vi "Solve1.vi"(8 "Error In":errorcluster, 11 "object in":refnum<class "2024_12.lvclass">) -> (0 "Error Out":errorcluster, 2 "Result":u64, 3 "object out":refnum<class "2024_12.lvclass">)   [LabVIEW 2023, in "2024_12.lvclass"]
uses:
  2024_12.lvclass
  2024_12.lvclass/2024_12.ctl
  f444b186-b13a-4318-b9c4-f3d0cdaa4562.vi
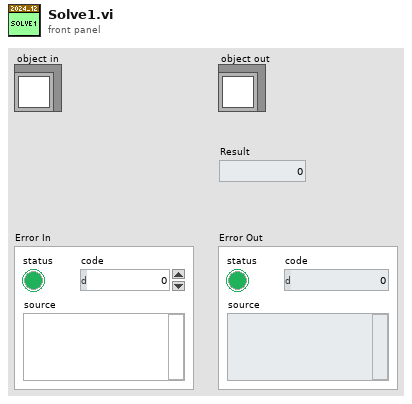
[diagram p1: front panel]
types:
  T1 = cluster{u8, cluster{i32, i32}, "PixelsFound":cluster{"x":i32, "y":i32}[]}
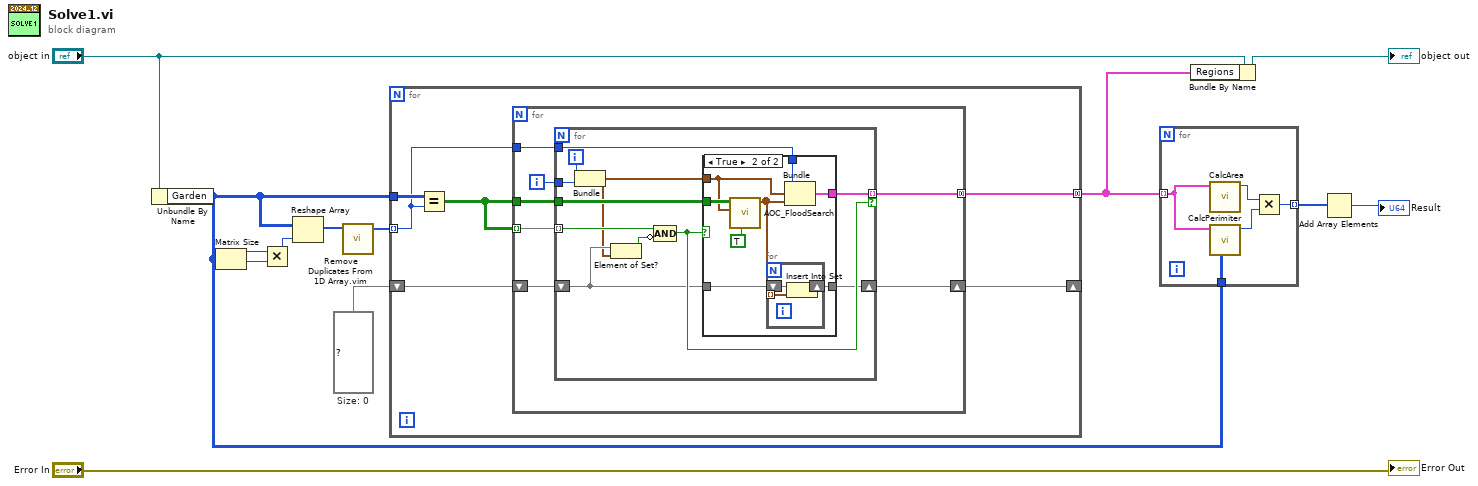
[diagram p0: block diagram]
diagram:
  w6 = set{cluster{"x":i32, "y":i32}} {}  # Size: 0
  n1 = Unbundle By Name("object in") -> ("Garden"=w3:u8[][])
  n2 = Matrix Size(0:w3) -> (1:w11:i32, 2:w10:i32)
  n3 = Multiply(x=w11, y=w10) -> (x*y=w9:i32)
  n4 = Reshape Array(w3, w9) -> (w8:u8[])
  n5 = call "Remove Duplicates From 1D Array.vim"("array"=w8) -> ("array with duplicates removed"=w7:u8[])  [unwired: 10 in]
  n6 = for {
    tunnel: w3 -> [w19]
    tunnel: w7 -> [w17] mode=indexing
    shift-right: [w15] -> _
    shift-left: w6 -> [w16]
    tunnel: [w14] -> w1 mode=concatenating
    n7 = Equal?(x=w19, y=w17) -> (x = y?=w18:bool[][])
    n8 = for {
      tunnel: w18 -> [w26]
      tunnel: w18 -> [w25] mode=indexing
      tunnel: w17 -> [w23]
      shift-right: [w21] -> w15
      shift-left: w16 -> [w22]
      tunnel: [w20] -> w14 mode=concatenating
      i -> [w24]
      n9 = for {
        tunnel: w26 -> [w37]
        tunnel: w25 -> [w36] mode=indexing
        tunnel: w24 -> [w35]
        tunnel: [w33] -> w20 mode=indexing if=w31
        tunnel: w23 -> [w32]
        shift-right: [w30] -> w21
        shift-left: w22 -> [w29]
        i -> [w34]
        n10 = Bundle(w34, w35) -> (w28:cluster{i32, i32})  [unwired: 1 in]
        n11 = Element of Set?(10:w28, 11:w29) -> (3:w27:bool)
        n12 = Compound Arithmetic op=AND(w36, invert w27) -> (w31:bool)
        n13 = case shown="True" w31 {
          tunnel: w37 -> [_ w46]
          tunnel: w28 -> [_ w45]
          tunnel: [_ w44] -> w33
          tunnel: w32 -> [_ w43]
          tunnel: w29 -> [w38 w42]
          tunnel: [w38 w41] -> w30
          frame False {
          }
          frame True {
            n14 = call "AOC_FloodSearch.vi"("4 (T) or 8 (F)"=TRUE, "Start Position"=w45, "DataIn"=w46) -> ("PixelsFound"=w40:cluster{"x":i32, "y":i32}[])  [unwired: 5 in, 3 out]
            n15 = for {
              shift-right: [w48] -> w41
              shift-left: w42 -> [w49]
              tunnel: w40 -> [w47] mode=indexing
              n16 = Insert Into Set(10:w47, 11:w49) -> (3:w48:set{cluster{"x":i32, "y":i32}})  [unwired: 1 out]
            }
            n17 = Bundle(w43, w45, "PixelsFound"=w40) -> (w44:T1)  [unwired: 1 in]
          }
        }
      }
    }
  }
  n18 = for {
    tunnel: w1 -> [w54] mode=indexing
    tunnel: [w52] -> w5 mode=indexing
    tunnel: w3 -> [w51]
    n19 = call "CalcArea.vi"("Cluster"=w54) -> ("Numeric"=w50:u64)  [unwired: 10 in]
    n20 = call "CalcPerimiter.vi"("Garden"=w51, "Cluster"=w54) -> ("Numeric"=w53:u64)  [unwired: 9 in]
    n21 = Multiply(x=w50, y=w53) -> (x*y=w52:u64)
  }
  n22 = Bundle By Name(cluster="object in", "Regions"=w1) -> (→"object out":refnum<class "2024_12.lvclass">)
  n23 = Add Array Elements(numeric array=w5) -> (sum=→"Result":u64)
  "Error Out" <- "Error In"
